vi "Check PassWord.vi"(8 "error in (no error)":errorcluster, 9 "Permission":T1, 10 "Caller ActorQName":string, 11 "CallActorCenter in":refnum<class "CallActorCenter.lvclass">) -> (0 "error out":errorcluster, 3 "CallActorCenter out":refnum<class "CallActorCenter.lvclass">)   [LabVIEW 2021, in "CallActorCenter.lvclass"]
uses:
  CallActorCenter.lvclass
  C:/Program Files (x86)/National Instruments/LabVIEW 2021/user.lib/John_Lib/AbstractActorTemplate/AbstractActorTemplate/UIActorTop.lvclass
  <userlib>/John_Lib/Interfaces/CheckPassWord/Permission.ctl
  <userlib>/John_Lib/Interfaces/CheckPassWord Messages/Check PassWord Msg/Check PassWord Msg.lvclass/Check PassWord Msg.ctl
  <vilib>/ActorFramework/Message Enqueuer/Message Enqueuer.lvclass/Message Enqueuer.ctl
  <vilib>/ActorFramework/Message Enqueuer/Enqueue.vi
  <userlib>/John_Lib/Interfaces/CheckPassWord Messages/Check PassWord Msg/Check PassWord Msg.lvclass
  C:/Program Files (x86)/National Instruments/LabVIEW 2021/vi.lib/ActorFramework/Message/Message.lvclass
  <vilib>/ActorFramework/Message Priority Queue/Priority Enqueue.vi
  CallActorCenter.lvclass/CallActorCenter.ctl
  <userlib>/John_Lib/AbstractActorTemplate/AbstractActorTemplate/UIActorTop.lvclass
  <userlib>/John_Lib/Interfaces/CheckPassWord/CheckPassWord.lvclass
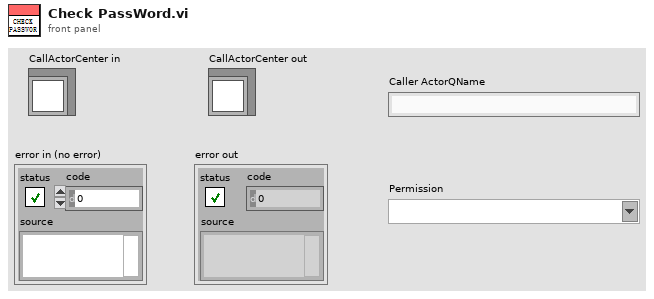
[diagram p1: front panel]
types:
  T1 = typedef "CheckPassWord.lvlib/CheckPassWord.lvclass/Permission.ctl" = string
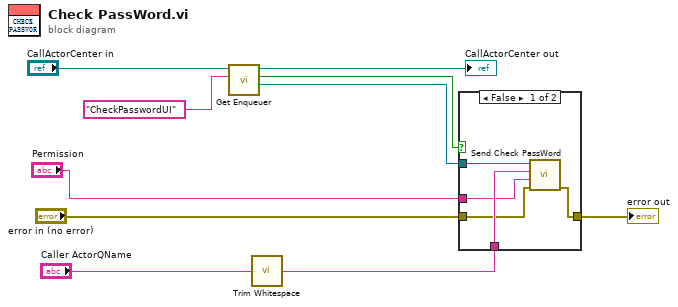
[diagram p0: block diagram]
diagram:
  n1 = call <userlib>:"Get Enqueuer.vi"("ActorQName"="CheckPasswordUI", "UIActorTop in"="CallActorCenter in") -> ("Nested Actor's Enqueuer"=w3:refnum<class "Message Enqueuer.lvclass">, "key not found?"=w2:bool, "UIActorTop out"=→"CallActorCenter out":refnum<class "CallActorCenter.lvclass">)  [unwired: 6 in, 1 out]
  n2 = call <vilib>:"Trim Whitespace.vi"("string"="Caller ActorQName") -> ("trimmed string"=w10:string)  [unwired: 1 in]
  n3 = case shown="False" w2 {
    tunnel: [w12 w16] -> w6
    tunnel: "error in (no error)" -> [w13 w16]
    tunnel: w3 -> [w15 _]
    tunnel: w10 -> [w14 _]
    tunnel: "Permission" -> [w11 _]
    frame False {
      n4 = call <userlib>:"Send Check PassWord.vi"("error in (no error)"=w13, "Permission"=w11, "Caller ActorQName"=w14, "Message Enqueuer"=w15) -> ("error out"=w12:errorcluster)  [unwired: 6 in, 1 out]
    }
    frame True {
    }
  }
  "error out" <- w6
